vi "Launch.vi"(8 "error in (no error)":errorcluster caption="entrée d'erreur (pas d'erreur)", 11 "Process (Default) en entrée":refnum<class "Process (Default).lvclass">) -> (0 "error out":errorcluster caption="sortie d'erreur", 3 "Process (Default) en sortie":refnum<class "Process (Default).lvclass">)   [LabVIEW 2020, in "Library Instrument & Equipement.lvlib" / "Process (Default).lvclass"]
uses:
  Process (Default).lvclass
  Process (Default).lvclass/Process (Default).ctl
  dccef7bf-8787-4f97-810e-f0d14b49e394.vi
  Variable dispatch.vi
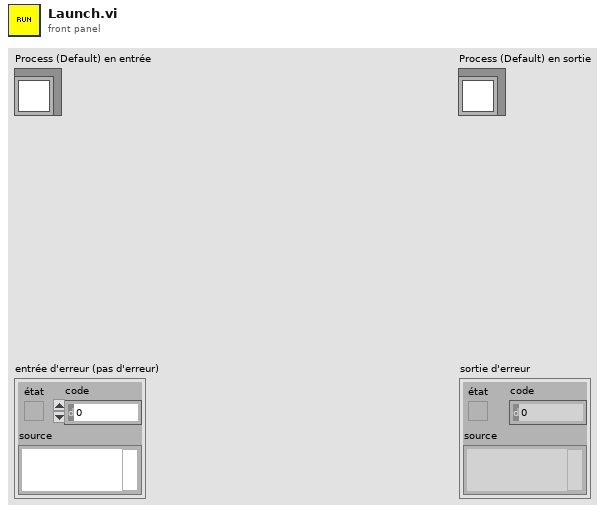
[diagram p1: front panel]
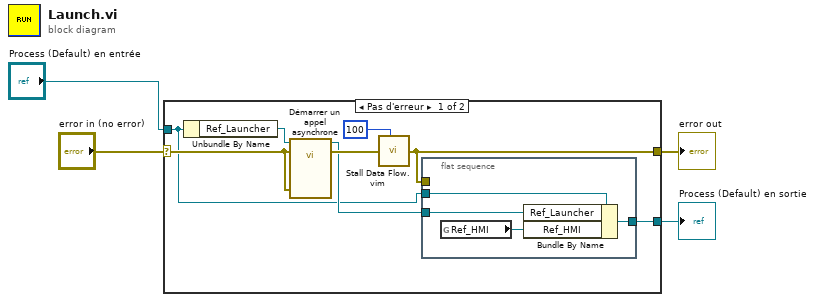
[diagram p0: block diagram]
diagram:
  n1 = case shown="Pas d'erreur" "error in (no error)" {
    selector: "error in (no error)" -> [w8 w18]
    tunnel: [w7 w18] -> w3
    tunnel: [w5 w17] -> w1
    tunnel: "Process (Default) en entrée" -> [w6 w17]
    frame No Error {
      n2 = Unbundle By Name(w6) -> ("Ref_Launcher"=w9:refnum<vi>)
      n3 = call-by-ref "Démarrer un appel asynchrone"(reference=w9, error in=w8, 8:"error in (no error)"=w8) -> (reference out=w10:refnum<vi>, error out=w12:errorcluster)  [unwired: 10 in, 1 out]
      n4 = call "Stall Data Flow.vim"("value in"=w12, "milliseconds to wait"=u32 100) -> ("value out"=w7:errorcluster)  [unwired: 1 out]
      n5 = flat-sequence {
        tunnel: [w16] -> w5
        tunnel: w6 -> [w15]
        tunnel: w10 -> [w14]
        tunnel: w7 -> [_]
        frame #0 {
          n6 = global read "Variable dispatch.vi" "Ref_HMI"() -> (w13:refnum<vi>)
          n7 = Bundle By Name(cluster=w15, "Ref_Launcher"=w14, "Ref_HMI"=w13) -> (w16:refnum<class "Process (Default).lvclass">)
        }
      }
    }
    frame Error {
    }
  }
  "error out" <- w3
  "Process (Default) en sortie" <- w1
